vi "read ocean (SubVI).vi"(10 "Enable Strobe (Disabled)":bool, 11 "VISA Refnum in":refnum<visa-resource-name>) -> (2 "Spectrum by Pixels":dbl[](array[numeric]), 3 "Wavelength (nm)":dbl[](array[numeric]))   [LabVIEW 2019]
uses:
  C/Program Files (x86)/National Instruments/LabVIEW 2020/instr.lib/Ocean Optics 2000 4000/Ocean Optics 2000 4000.lvlib
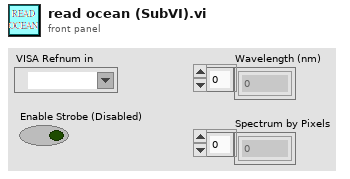
[diagram p1: front panel]
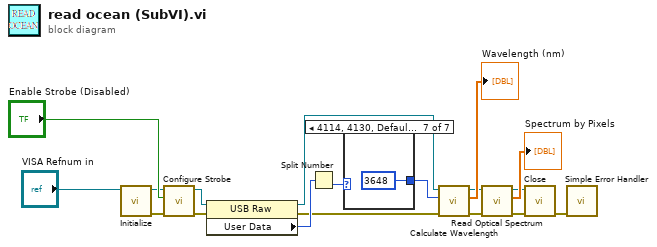
[diagram p0: block diagram]
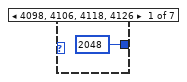
[diagram p2: hidden frame]
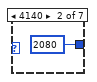
[diagram p3: hidden frame]
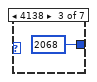
[diagram p4: hidden frame]
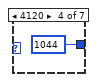
[diagram p5: hidden frame]
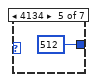
[diagram p6: hidden frame]
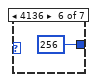
[diagram p7: hidden frame]
diagram:
  n1 = call "Initialize.vi"("VISA resource name"="VISA Refnum in") -> ("error out"=w13:errorcluster, "VISA resource name out"=w14:refnum<visa-resource-name>)  [unwired: 2 in, 7 out]
  n2 = call "Configure Strobe.vi"("error in (no error)"=w13, "Enable Strobe (Disabled)"="Enable Strobe (Disabled)", "VISA resource name"=w14) -> ("error out"=w3:errorcluster, "VISA resource name out"=w4:refnum<visa-resource-name>)  [unwired: 7 out]
  n3 = property class="USB Raw"(reference=w4, error in=w3) -> (reference out=w6:refnum<visa-resource-name>, error out=w5:errorcluster, "User Data"=w9:u32)
  n4 = Split Number(x=w9) -> (lo(x)=w8:u16)  [unwired: 1 out]
  n5 = case shown="4114, 4130, Default" w8 {
    tunnel: [2048 ("Number of Pixels (3840)") 2080 ("Number of Pixels (3840)") 2068 ("Number of Pixels (3840)") 1044 ("Number of Pixels (3840)") 512 ("Number of Pixels (3840)") 256 ("Number of Pixels (3840)") 3648 ("Number of Pixels (3840)")] -> w7
    frame 4098, 4106, 4118, 4126 {
    }
    frame 4140 {
    }
    frame 4138 {
    }
    frame 4120 {
    }
    frame 4134 {
    }
    frame 4136 {
    }
    frame 4114, 4130, Default {
    }
  }
  n6 = call "Calculate Wavelength.vi"("error in (no error)"=w5, "Number of Pixels (3648)"=w7, "VISA resource name"=w6) -> ("error out"=w1:errorcluster, "Wavelength (nm)"=→"Wavelength (nm)":dbl[], "VISA resource name out"=w2:refnum<visa-resource-name>)  [unwired: 6 out]
  n7 = call "Read Optical Spectrum.vi"("error in (no error)"=w1, "VISA resource name"=w2) -> ("error out"=w11:errorcluster, "Spectrum by Pixels"=→"Spectrum by Pixels":dbl[], "VISA resource name out"=w12:refnum<visa-resource-name>)  [unwired: 7 out]
  n8 = call "Close.vi"("error in (no error)"=w11, "VISA resource name"=w12) -> ("error out"=w10:errorcluster)  [unwired: 9 out]
  n9 = call <vilib>:"Simple Error Handler.vi"("error in (no error)"=w10) -> ()  [unwired: 1 in, 8 out]
